vi "Average BScan.vi"(11 "B-Scan In":u16[][](array[numeric])) -> (3 "Averaged BScan":dbl[](graph))   [LabVIEW 2014]
panel:
  out "Intensity Graph":sgl[][](graph)
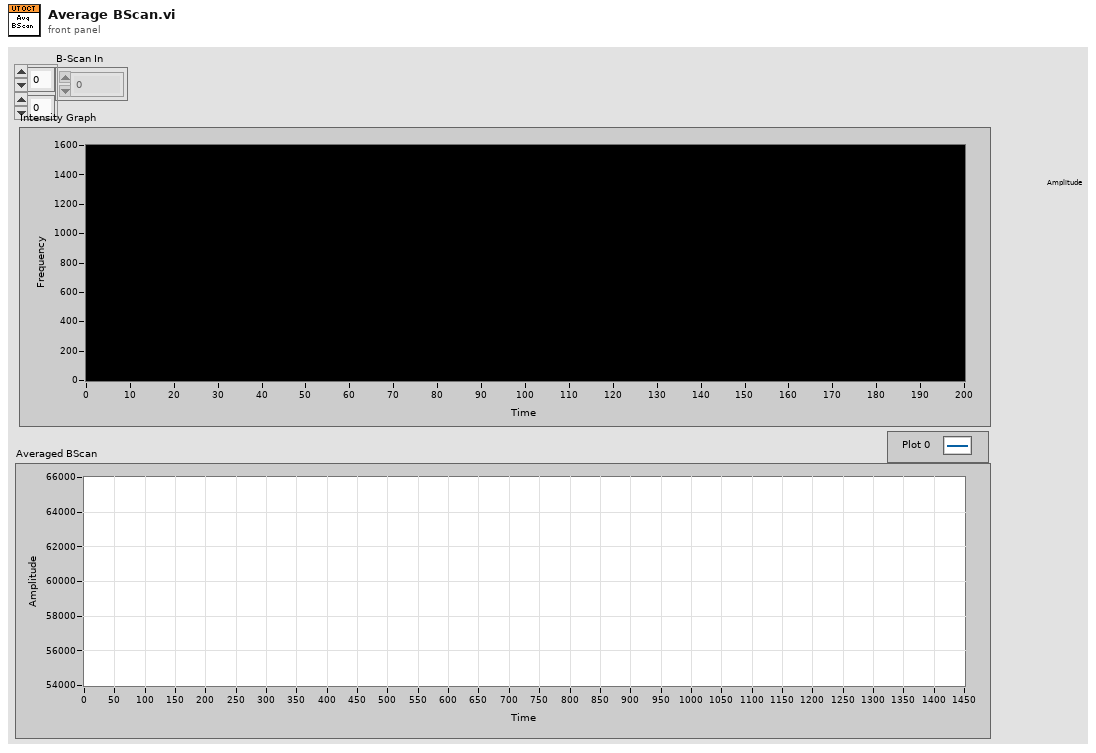
[diagram p1: front panel]
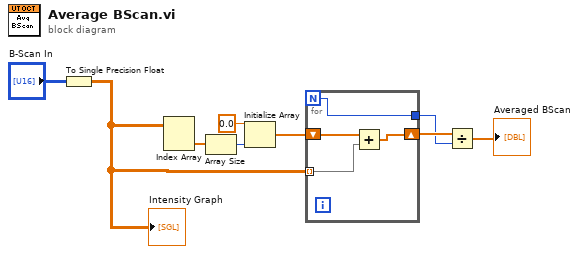
[diagram p0: block diagram]
diagram:
  n1 = To Single Precision Float(number="B-Scan In") -> (single precision float=w1:sgl[][])
  "Intensity Graph" <- w1
  n2 = Index Array(array=w1) -> (element=w7:sgl[])  [unwired: 2 in]
  n3 = Array Size(array=w7) -> (size(s)=w8:i32)
  n4 = Initialize Array(0.0 ("element"), w8) -> (w5:dbl[])
  n5 = for {
    N -> [w10]
    shift-right: [w11] -> w4
    shift-left: w5 -> [w13]
    tunnel: w1 -> [w12] mode=indexing
    tunnel: [w10] -> w3
    n6 = Add(x=w13, y=w12) -> (x+y=w11:dbl[])
  }
  n7 = Divide(x=w4, y=w3) -> (x/y=→"Averaged BScan":dbl[])
